vi "Write Min Depth Message.vi"(8 "error in (no error)":errorcluster, 10 "Min Depth":u8, 11 "AIP Set Min Depth Message in":refnum<class "AIP Set Min Depth Message.lvclass">) -> (0 "error out":errorcluster, 3 "AIP Set Min Depth Message out":refnum<class "AIP Set Min Depth Message.lvclass">)   [LabVIEW 2015, in "RDS Child Messages.lvlib" / "AIP Set Min Depth Message.lvclass"]
uses:
  AIP Set Min Depth Message.lvclass
  AIP Set Min Depth Message.lvclass/AIP Set Min Depth Message.ctl
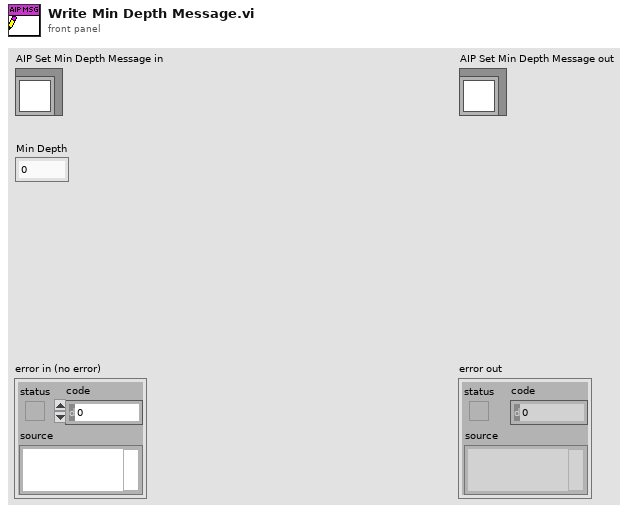
[diagram p1: front panel]
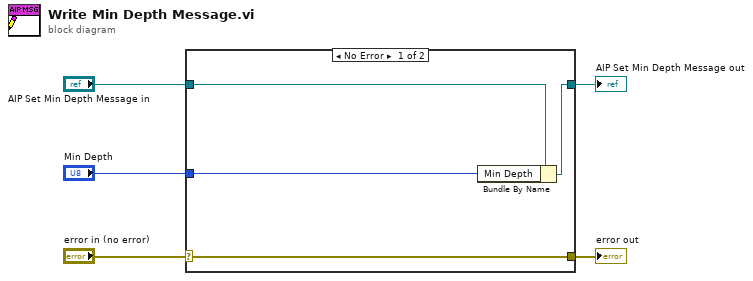
[diagram p0: block diagram]
diagram:
  n1 = case shown="No Error" "error in (no error)" {
    selector: "error in (no error)" -> [w9 w10]
    tunnel: [w9 w10] -> w4
    tunnel: [w7 w11] -> w2
    tunnel: "AIP Set Min Depth Message in" -> [w8 w11]
    tunnel: "Min Depth" -> [w6 _]
    frame No Error {
      n2 = Bundle By Name(cluster=w8, "Min Depth"=w6) -> (w7:refnum<class "AIP Set Min Depth Message.lvclass">)
    }
    frame Error {
    }
  }
  "error out" <- w4
  "AIP Set Min Depth Message out" <- w2
